vi "Formula_Node.vi"() -> ()   [LabVIEW 2017]
panel:
  out "Tf":dbl
  in  "Tc":dbl
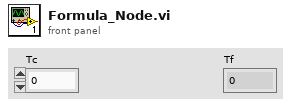
[diagram p1: front panel]
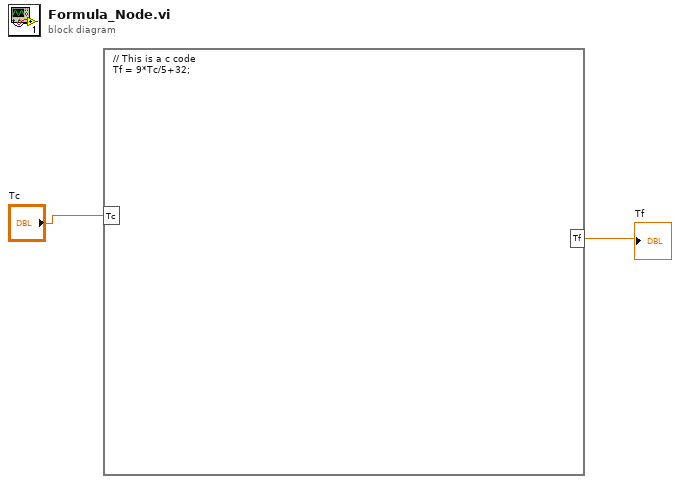
[diagram p0: block diagram]
diagram:
  n1 = formula code="// This is a c code\nTf = 9*Tc/5+32;"("Tc"="Tc") -> ("Tf"=→"Tf":dbl)
